vi "IMU2JointAngles.vi"(4 "ResetStandPos":bool, 6 "SetStandPos":bool, 7 "JointAngleDir":dbl[](array[numeric]), 8 "error in (no error)":errorcluster, 9 "LockHipAbduction(F)":bool, 10 "LockHipRotation(T)":bool=TRUE, 11 "IMU in (rad)":dbl[][](array[numeric])) -> (0 "error out":errorcluster, 2 "StandPos":dbl[](array[numeric]), 3 "Joint Angles (rad)":dbl[](array[numeric]))   [LabVIEW 2016]
uses:
  <vilib>/Analysis/Matrix/Datatypes/RealMatrix.ctl
  <vilib>/Analysis/BLAS.llb/LV_Transpose.ctl
  <vilib>/Analysis/coordinate.llb/Euler Rotation Order.ctl
  <vilib>/Analysis/BLAS.llb/dgemm - General Matrix-Matrix Product (DBL).vi
  <vilib>/Analysis/NI_AALPro.lvlib
  <vilib>/Analysis/NI_AALBLAS.lvlib
  <vilib>/Analysis/Matrix/NI_Matrix.lvlib
panel:
  out "R_CtoS_Shank":dbl[][](array[numeric])=[[0.0, 0.0, -1.0], [1.0, 0.0, 0.0], [0.0, -1.0, 0.0]]
  out "R_CtoS_Thigh":dbl[][](array[numeric])=[[0.0, 0.0, -1.0], [1.0, 0.0, 0.0], [0.0, -1.0, 0.0]]
  out "R_CtoS_Hip":dbl[][](array[numeric])=[[0.0, 0.0, -1.0], [1.0, 0.0, 0.0], [0.0, -1.0, 0.0]]
  in  "UseStandPos(T)":bool=TRUE
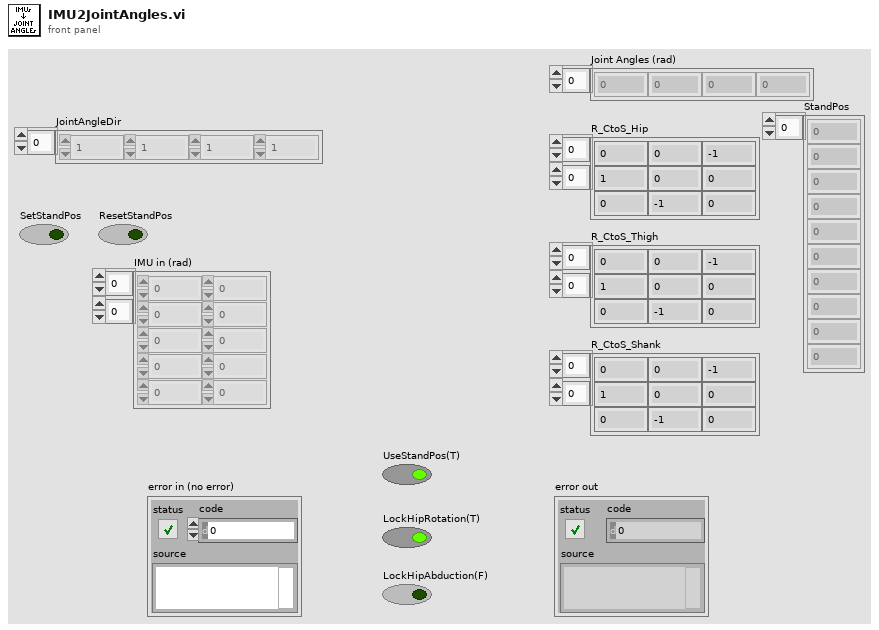
[diagram p1: front panel]
types:
  T1 = typedef "NI_Matrix.lvlib/RealMatrix.ctl" = dbl[][]
  T2 = typedef "NI_AALPro.lvlib/Euler Rotation Order.ctl" = u16
  T3 = typedef "NI_AALBLAS.lvlib/LV_Transpose.ctl" = i32
  T4 = cluster{"IMU in (rad)[0]":dbl, "IMU in (rad)[1]":dbl, "IMU in (rad)[2]":dbl}
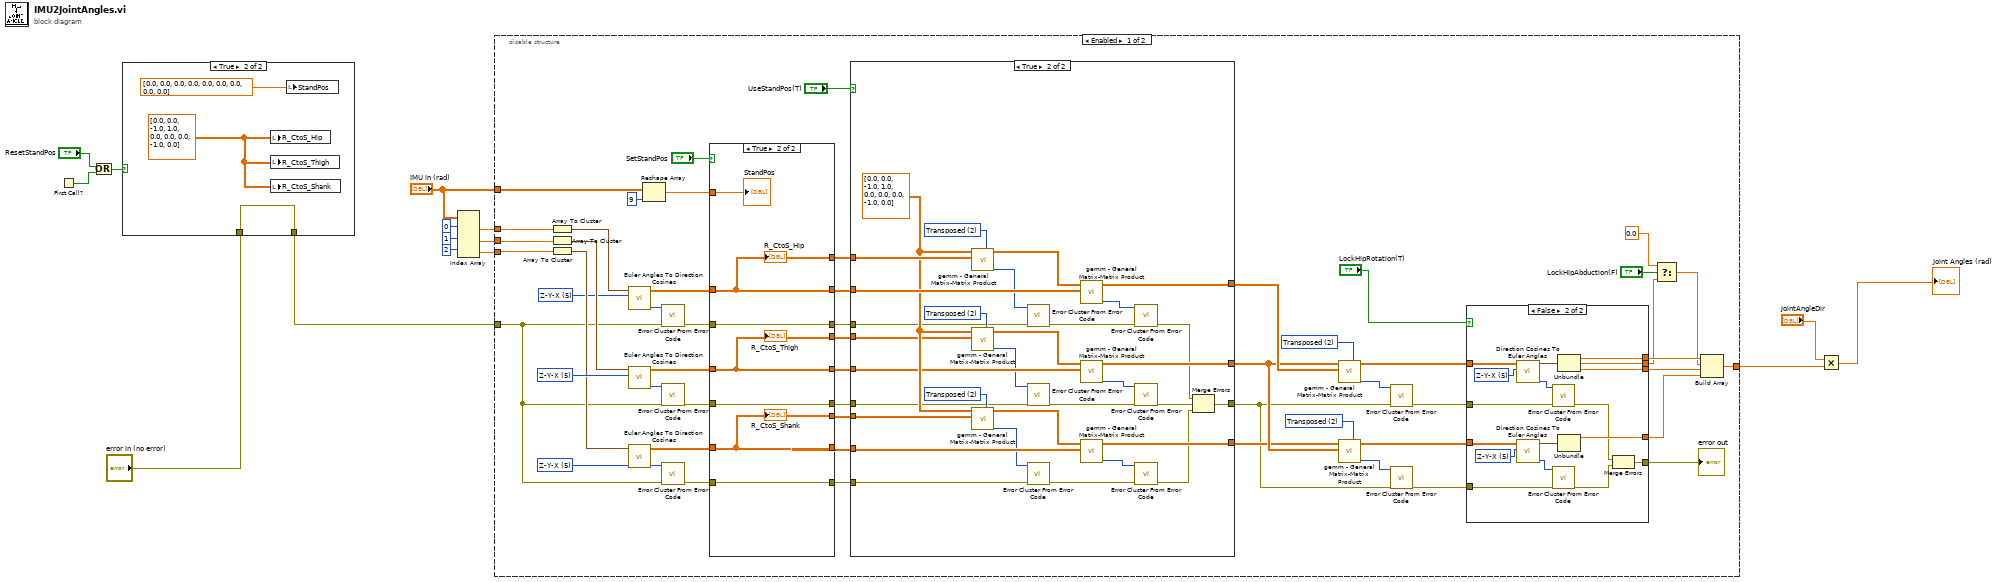
[diagram p0: block diagram]
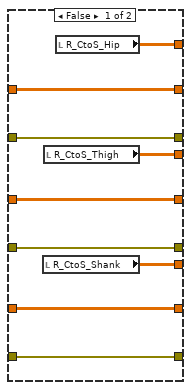
[diagram p3: hidden frame]
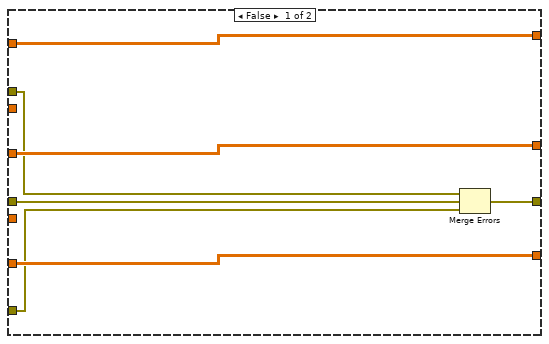
[diagram p4: hidden frame]
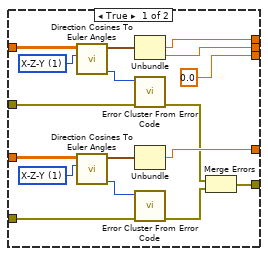
[diagram p5: hidden frame]
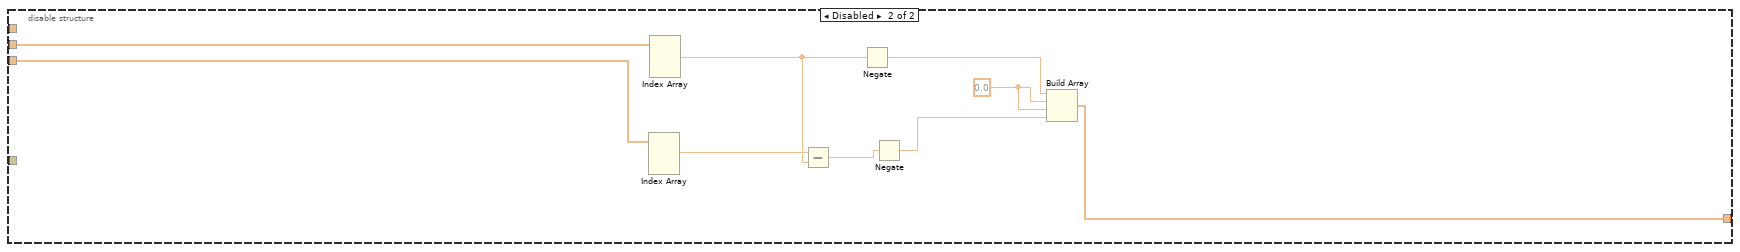
[diagram p6: hidden frame]
diagram:
  n1 = First Call?() -> (First Call?: T/F=w6:bool)
  n2 = Or(x="ResetStandPos", y=w6) -> (x .or. y?=w4:bool)
  n3 = case shown="True" w4 {
    tunnel: "error in (no error)" -> [w16 w18]
    tunnel: [w16 w18] -> w2
    frame False {
    }
    frame True {
      w19 = T1 [[0.0, 0.0, -1.0], [1.0, 0.0, 0.0], [0.0, -1.0, 0.0]] ("A")
      n4 = local write "R_CtoS_Hip"(w19) -> ()
      n5 = local write "R_CtoS_Thigh"(w19) -> ()
      n6 = local write "R_CtoS_Shank"(w19) -> ()
      n7 = local write "StandPos"(dbl[] [0.0, 0.0, 0.0, 0.0, 0.0, 0.0, 0.0, 0.0, 0.0] ("ZeroOrient")) -> ()
    }
  }
  n8 = Index Array(array="IMU in (rad)", index (row) #1=0 ("index (row)"), index (row) #2=1 ("index (row)"), index (row) #3=2 ("index (row)")) -> (element #1=w7:dbl[], element #2=w9:dbl[], element #3=w8:dbl[])  [unwired: 3 in]
  n9 = disable-structure shown="Enabled" {
    disable-tunnel: w9 -> [w24 w172]
    disable-tunnel: w8 -> [w23 w171]
    disable-tunnel: [w70 w165] -> w13
    disable-tunnel: w7 -> [w25 _]
    disable-tunnel: w2 -> [w36 _]
    disable-tunnel: "IMU in (rad)" -> [w22 _]
    frame Enabled {
      w63 = T2 5 items=["X-Y-Z", "X-Z-Y", "Y-X-Z", "Y-Z-X", "Z-X-Y", "Z-Y-X", "X-Y-X", "X-Z-X", "Y-X-Y", "Y-Z-Y", "Z-X-Z", "Z-Y-Z"] ("rotation order")
      w62 = T3 2 items=["Direct", "Conjugated & Transposed", "Transposed"] ("operation B")
      w61 = T3 2 items=["Direct", "Conjugated & Transposed", "Transposed"] ("operation B")
      w72 = T2 5 items=["X-Y-Z", "X-Z-Y", "Y-X-Z", "Y-Z-X", "Z-X-Y", "Z-Y-X", "X-Y-X", "X-Z-X", "Y-X-Y", "Y-Z-Y", "Z-X-Z", "Z-Y-Z"] ("rotation order")
      w74 = T2 5 items=["X-Y-Z", "X-Z-Y", "Y-X-Z", "Y-Z-X", "Z-X-Y", "Z-Y-X", "X-Y-X", "X-Z-X", "Y-X-Y", "Y-Z-Y", "Z-X-Z", "Z-Y-Z"] ("rotation order")
      n10 = Array To Cluster(array=w25) -> (cluster=w68:T4)
      n11 = Array To Cluster(array=w24) -> (cluster=w73:T4)
      n12 = Array To Cluster(array=w23) -> (cluster=w71:T4)
      n13 = call <vilib>:"Euler Angles To Direction Cosines.vi"("rotation order"=w63, "Euler Angles"=w68) -> ("error"=w45:i32, "Direction Cosines"=w46:dbl[][])  [unwired: 8 in]
      n14 = call <vilib>:"Euler Angles To Direction Cosines.vi"("rotation order"=w74, "Euler Angles"=w73) -> ("error"=w44:i32, "Direction Cosines"=w48:dbl[][])  [unwired: 8 in]
      n15 = call <vilib>:"Euler Angles To Direction Cosines.vi"("rotation order"=w72, "Euler Angles"=w71) -> ("error"=w43:i32, "Direction Cosines"=w53:dbl[][])  [unwired: 8 in]
      n16 = Reshape Array(w22, 9 ("dimension size")) -> (w20:dbl[])
      n17 = call <vilib>:"Error Cluster From Error Code.vi"("error in (no error)"=w36, "error code (0)"=w45) -> ("error out"=w42:errorcluster)  [unwired: 7 in]
      n18 = call <vilib>:"Error Cluster From Error Code.vi"("error in (no error)"=w36, "error code (0)"=w44) -> ("error out"=w40:errorcluster)  [unwired: 7 in]
      n19 = call <vilib>:"Error Cluster From Error Code.vi"("error in (no error)"=w36, "error code (0)"=w43) -> ("error out"=w37:errorcluster)  [unwired: 7 in]
      n20 = case shown="True" "SetStandPos" {
        tunnel: [w80 w88] -> w54
        tunnel: w53 -> [w80 w88]
        tunnel: [w83 w90] -> w52
        tunnel: [w82 w89] -> w51
        tunnel: [w81 w88] -> w50
        tunnel: [w79 w89] -> w49
        tunnel: w48 -> [w79 w89]
        tunnel: [w78 w90] -> w47
        tunnel: w46 -> [w78 w90]
        tunnel: w42 -> [w77 w87]
        tunnel: [w77 w87] -> w41
        tunnel: w40 -> [w76 w86]
        tunnel: [w76 w86] -> w39
        tunnel: [w75 w85] -> w38
        tunnel: w37 -> [w75 w85]
        tunnel: w20 -> [_ w84]
        frame False {
          n21 = local read "R_CtoS_Shank"() -> (w81:dbl[][])
          n22 = local read "R_CtoS_Thigh"() -> (w82:dbl[][])
          n23 = local read "R_CtoS_Hip"() -> (w83:dbl[][])
        }
        frame True {
          "R_CtoS_Hip" <- w90
          "R_CtoS_Thigh" <- w89
          "R_CtoS_Shank" <- w88
          "StandPos" <- w84
        }
      }
      n24 = case shown="True" "UseStandPos(T)" {
        tunnel: w47 -> [w97 w129]
        tunnel: [w97 w126] -> w59
        tunnel: [w96 w124] -> w58
        tunnel: w49 -> [w96 w114]
        tunnel: w54 -> [w95 w121]
        tunnel: [w95 w120] -> w57
        tunnel: w52 -> [_ w125]
        tunnel: w51 -> [_ w116]
        tunnel: w50 -> [_ w115]
        tunnel: w41 -> [w93 w104]
        tunnel: w39 -> [w92 w103]
        tunnel: w38 -> [w91 w102]
        tunnel: [w94 w98] -> w35
        frame False {
          n25 = Merge Errors(w93, w92, w91) -> (w94:errorcluster)
        }
        frame True {
          w117 = T3 2 items=["Direct", "Conjugated & Transposed", "Transposed"] ("operation B")
          w118 = T3 2 items=["Direct", "Conjugated & Transposed", "Transposed"] ("operation B")
          w127 = T3 2 items=["Direct", "Conjugated & Transposed", "Transposed"] ("operation B")
          w119 = T1 [[0.0, 0.0, -1.0], [1.0, 0.0, 0.0], [0.0, -1.0, 0.0]] ("A")
          n26 = call-poly <vilib>:"gemm - General Matrix-Matrix Product.vi"("operation B"=w127, "B"=w125, "A"=w119) -> ("error"=w113:i32, "dgemm"=w128:T1)  [unwired: 7 in]
          n27 = call-poly <vilib>:"gemm - General Matrix-Matrix Product.vi"("operation B"=w118, "B"=w116, "A"=w119) -> ("error"=w112:i32, "dgemm"=w123:T1)  [unwired: 7 in]
          n28 = call-poly <vilib>:"gemm - General Matrix-Matrix Product.vi"("operation B"=w117, "B"=w115, "A"=w119) -> ("error"=w111:i32, "dgemm"=w122:T1)  [unwired: 7 in]
          n29 = call <vilib>:"Error Cluster From Error Code.vi"("error in (no error)"=w104, "error code (0)"=w113) -> ("error out"=w109:errorcluster)  [unwired: 7 in]
          n30 = call <vilib>:"Error Cluster From Error Code.vi"("error in (no error)"=w103, "error code (0)"=w112) -> ("error out"=w107:errorcluster)  [unwired: 7 in]
          n31 = call <vilib>:"Error Cluster From Error Code.vi"("error in (no error)"=w102, "error code (0)"=w111) -> ("error out"=w105:errorcluster)  [unwired: 7 in]
          n32 = call-poly <vilib>:"gemm - General Matrix-Matrix Product.vi"("B"=w129, "A"=w128) -> ("error"=w110:i32, "dgemm"=w126:T1)  [unwired: 8 in]
          n33 = call-poly <vilib>:"gemm - General Matrix-Matrix Product.vi"("B"=w114, "A"=w123) -> ("error"=w108:i32, "dgemm"=w124:T1)  [unwired: 8 in]
          n34 = call-poly <vilib>:"gemm - General Matrix-Matrix Product.vi"("B"=w121, "A"=w122) -> ("error"=w106:i32, "dgemm"=w120:T1)  [unwired: 8 in]
          n35 = call <vilib>:"Error Cluster From Error Code.vi"("error in (no error)"=w109, "error code (0)"=w110) -> ("error out"=w101:errorcluster)  [unwired: 7 in]
          n36 = call <vilib>:"Error Cluster From Error Code.vi"("error in (no error)"=w107, "error code (0)"=w108) -> ("error out"=w100:errorcluster)  [unwired: 7 in]
          n37 = call <vilib>:"Error Cluster From Error Code.vi"("error in (no error)"=w105, "error code (0)"=w106) -> ("error out"=w99:errorcluster)  [unwired: 7 in]
          n38 = Merge Errors(w101, w100, w99) -> (w98:errorcluster)
        }
      }
      n39 = call-poly <vilib>:"gemm - General Matrix-Matrix Product.vi"("operation B"=w62, "B"=w59, "A"=w58) -> ("error"=w34:i32, "dgemm"=w64:T1)  [unwired: 7 in]
      n40 = call-poly <vilib>:"gemm - General Matrix-Matrix Product.vi"("operation B"=w61, "B"=w58, "A"=w57) -> ("error"=w33:i32, "dgemm"=w69:T1)  [unwired: 7 in]
      n41 = call <vilib>:"Error Cluster From Error Code.vi"("error in (no error)"=w35, "error code (0)"=w34) -> ("error out"=w32:errorcluster)  [unwired: 7 in]
      n42 = call <vilib>:"Error Cluster From Error Code.vi"("error in (no error)"=w35, "error code (0)"=w33) -> ("error out"=w31:errorcluster)  [unwired: 7 in]
      n43 = case shown="False" "LockHipRotation(T)" {
        tunnel: [w139 w161] -> w29
        tunnel: w69 -> [w144 w160]
        tunnel: [w140 w159] -> w67
        tunnel: [0.0 ("psi") w158] -> w66
        tunnel: [w137 w157] -> w65
        tunnel: w64 -> [w143 w156]
        tunnel: w32 -> [w135 w152]
        tunnel: w31 -> [w133 w150]
        tunnel: [w130 w147] -> w30
        frame True {
          w142 = T2 1 items=["X-Y-Z", "X-Z-Y", "Y-X-Z", "Y-Z-X", "Z-X-Y", "Z-Y-X", "X-Y-X", "X-Z-X", "Y-X-Y", "Y-Z-Y", "Z-X-Z", "Z-Y-Z"] ("rotation order")
          w146 = T2 1 items=["X-Y-Z", "X-Z-Y", "Y-X-Z", "Y-Z-X", "Z-X-Y", "Z-Y-X", "X-Y-X", "X-Z-X", "Y-X-Y", "Y-Z-Y", "Z-X-Z", "Z-Y-Z"] ("rotation order")
          n44 = call <vilib>:"Direction Cosines To Euler Angles.vi"("rotation order"=w142, "Direction Cosines"=w143) -> ("error"=w136:i32, "Euler Angles"=w141:cluster{"phi":dbl, "theta":dbl, "psi":dbl})  [unwired: 8 in]
          n45 = call <vilib>:"Direction Cosines To Euler Angles.vi"("rotation order"=w146, "Direction Cosines"=w144) -> ("error"=w134:i32, "Euler Angles"=w145:cluster{"phi":dbl, "theta":dbl, "psi":dbl})  [unwired: 8 in]
          n46 = Unbundle(w141) -> ("theta"=w140:dbl, "psi"=w139:dbl)  [unwired: 1 out]
          n47 = call <vilib>:"Error Cluster From Error Code.vi"("error in (no error)"=w135, "error code (0)"=w136) -> ("error out"=w131:errorcluster)  [unwired: 7 in]
          n48 = Unbundle(w145) -> ("theta"=w137:dbl)  [unwired: 2 out]
          n49 = call <vilib>:"Error Cluster From Error Code.vi"("error in (no error)"=w133, "error code (0)"=w134) -> ("error out"=w132:errorcluster)  [unwired: 7 in]
          n50 = Merge Errors(w131, w132) -> (w130:errorcluster)
        }
        frame False {
          w155 = T2 5 items=["X-Y-Z", "X-Z-Y", "Y-X-Z", "Y-Z-X", "Z-X-Y", "Z-Y-X", "X-Y-X", "X-Z-X", "Y-X-Y", "Y-Z-Y", "Z-X-Z", "Z-Y-Z"] ("rotation order")
          w163 = T2 5 items=["X-Y-Z", "X-Z-Y", "Y-X-Z", "Y-Z-X", "Z-X-Y", "Z-Y-X", "X-Y-X", "X-Z-X", "Y-X-Y", "Y-Z-Y", "Z-X-Z", "Z-Y-Z"] ("rotation order")
          n51 = call <vilib>:"Direction Cosines To Euler Angles.vi"("rotation order"=w155, "Direction Cosines"=w156) -> ("error"=w153:i32, "Euler Angles"=w154:cluster{"phi":dbl, "theta":dbl, "psi":dbl})  [unwired: 8 in]
          n52 = call <vilib>:"Direction Cosines To Euler Angles.vi"("rotation order"=w163, "Direction Cosines"=w160) -> ("error"=w151:i32, "Euler Angles"=w162:cluster{"phi":dbl, "theta":dbl, "psi":dbl})  [unwired: 8 in]
          n53 = call <vilib>:"Error Cluster From Error Code.vi"("error in (no error)"=w152, "error code (0)"=w153) -> ("error out"=w149:errorcluster)  [unwired: 7 in]
          n54 = call <vilib>:"Error Cluster From Error Code.vi"("error in (no error)"=w150, "error code (0)"=w151) -> ("error out"=w148:errorcluster)  [unwired: 7 in]
          n55 = Unbundle(w154) -> ("phi"=w159:dbl, "theta"=w161:dbl, "psi"=w158:dbl)
          n56 = Unbundle(w162) -> ("phi"=w157:dbl)  [unwired: 2 out]
          n57 = Merge Errors(w149, w148) -> (w147:errorcluster)
        }
      }
      "error out" <- w30
      n58 = Select(t=0.0, s="LockHipAbduction(F)", f=w29) -> (s? t:f=w28:dbl)
      n59 = Build Array(w67, w28, w66, w65) -> (w70:dbl[])
    }
    frame Disabled {
      w164 = 0.0 ("element")
      n60 = Index Array(array=w171) -> (element #1=w169:dbl)  [unwired: 3 in, 2 out]
      n61 = Index Array(array=w172) -> (element #1=w168:dbl)  [unwired: 3 in, 2 out]
      n62 = Subtract(x=w169, y=w168) -> (x-y=w167:dbl)
      n63 = Negate(x=w168) -> (-x=w170:dbl)
      n64 = Negate(x=w167) -> (-x=w166:dbl)
      n65 = Build Array(w170, w164, w164, w166) -> (w165:dbl[])
    }
  }
  n66 = Multiply(x="JointAngleDir", y=w13) -> (x*y=→"Joint Angles (rad)":dbl[])
